vi "FindCloseTagByNameC.vi"(6 "offset (0)":i32, 10 "close Tag":string, 11 "string":string) -> (1 "after close tag":string, 2 "match close tag":string, 3 "before close tag":string, 4 "offset past close tag":i32)   [LabVIEW 2017]
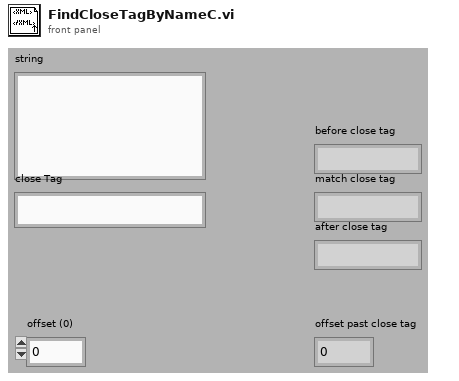
[diagram p1: front panel]
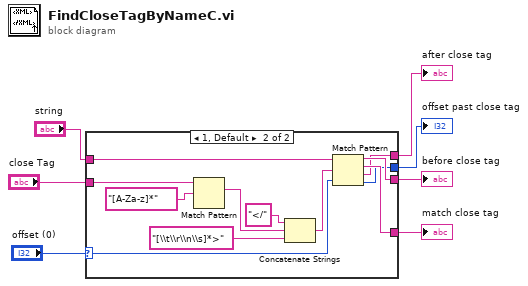
[diagram p0: block diagram]
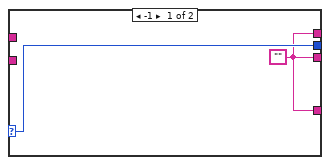
[diagram p2: hidden frame]
diagram:
  n1 = case shown="1, Default" "offset (0)" {
    selector: "offset (0)" -> [w9 w16]
    tunnel: "string" -> [_ w21]
    tunnel: "close Tag" -> [_ w10]
    tunnel: [w8 w20] -> w5
    tunnel: [w8 w19] -> w4
    tunnel: [w8 w18] -> w3
    tunnel: [w9 w17] -> w2
    frame -1 {
      w8 = ""
    }
    frame 1, Default {
      n2 = Match Pattern(string=w10, regular expression="[A-Za-z]*") -> (match substring=w11:string)  [unwired: 1 in, 3 out]
      n3 = Concatenate Strings("</" ("string"), w11, "[\\t\\r\\n\\s]*>" ("regular expression")) -> (w14:string)
      n4 = Match Pattern(string=w21, regular expression=w14, offset (0)=w16) -> (before substring=w20:string, match substring=w19:string, after substring=w18:string, offset past match=w17:i32)
    }
  }
  "before close tag" <- w5
  "match close tag" <- w4
  "after close tag" <- w3
  "offset past close tag" <- w2
